vi "BRig_RT__Case_Exp__recordAnalogInput__PortC__netstream.vi"(0 "input_buffer_dataAnalog":u16[][](array[numeric]), 1 "input_index":i32, 2 "input_iOccurence":u16, 3 "resetOccurrence":bool, 4 "input_dataCurrent":u16[](array[numeric]), 5 "input_empytyArray":u16[](array[numeric]), 6 "input_iState_start":T1, 7 "input_fifo_hdl":refnum<k33>, 8 "input_iState_end":T1, 9 "input_fifo_error":errorcluster, 10 "input_AI1":i16, 12 "input_AI0":i16) -> (11 "output_fifo_hdl":refnum<k33>, 13 "error out":errorcluster, 14 "output_buffer_dataAnalog":u16[][](array[numeric]), 15 "output_index":i32, 16 "output_iOccurrence":u16)   [LabVIEW 2014]
uses:
  myRIO_BRig_RT__Case_Exp_stateList.ctl
panel:
  out "error out 2":errorcluster
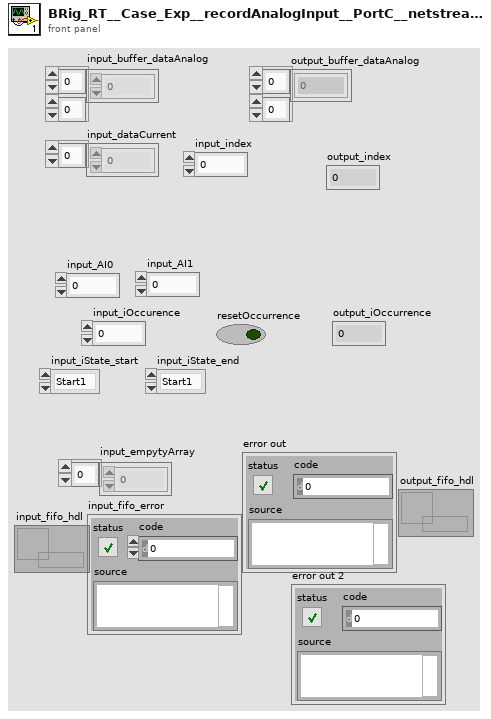
[diagram p1: front panel]
types:
  T1 = typedef "myRIO_BRig_RT__Case_Exp_stateList.ctl" = enum16{"Start1", "Start2", "Start3", "saveSettings1", "saveSettings2", "saveSettings3", "saveSettings4", "saveSettings_LC_ENL_l1", "saveSettings_LC_ENL_l2", "saveSettings_LC_Cue_l1", "saveSettings_LC_Cue_l2", "saveSettings6_LC_l1_Other", "SaveSettings6_LC_l2_Other", "setSettings_Audio", "setSettings_Laser", "initBlock_pre", "initBlock", "initBlock2", "initBlock_post", "initTrial_pre", "initTrial", "initTrial2", "initTrial3", "initTrial4", "initTrial_LC_ENL1", "initTrial_LC_Cue1", "initTrial_LC_Cue1_2", "initTrial_LC_Sel", "initTrial_post", "ENL1_pre", "ENL1", "ENL1_post", "ENL1Penalty_pre", "ENL1Penalty", "ENL2_pre", "ENL2", "ENL2Penalty_pre", "ENL2Penalty", "Cue1_pre", "Cue1", "Cue1_post", "Cue1Penalty_pre", "Cue1Penalty", "Cue2_pre", "Cue2", "Cue2Penalty_pre", "Cue2Penalty", "Selection_pre", "Selection", "Select_post", "SelectReward_pre", "SelectReward", "SelectRewardPost_pre", "SelectRewardPost", "SelectWrong_pre", "SelectWrong", "SelectWrong_post", "SelectTimeout_pre", "SelectTimeout", "SelectTimeout_post", "endTrial_pre", "endTrial1", "endTrial2", "endTrial3", "endTrial_post", "endBlock_pre", "endBlock", "endBlock_post", "endExp", "commConnect", "commUpload_pre", "commUpload_dataBlock", "commUpload_dataCurrent", "commUpload_dataExp", "commUpload_dataLC", "commUpload_dataTrial", "commUpload_post", "saveData_pre", "saveData_dataBlock", "saveData_dataCurrent", "saveData_dataExp", "saveData_dataLC", "saveData_dataTrial", "saveData_post", "empty_endBlock1", "empty_endBlock2", "empty_endTrial1", "empty_endTrial2", "empty_endTrial3", "empty_endTrial4", "empty_endTrial5", "dummyState", "dummyState_endBlock", "FreeReward_pre", "FreeReward", "FreeRewardPost_pre", "FreeRewardPost"}
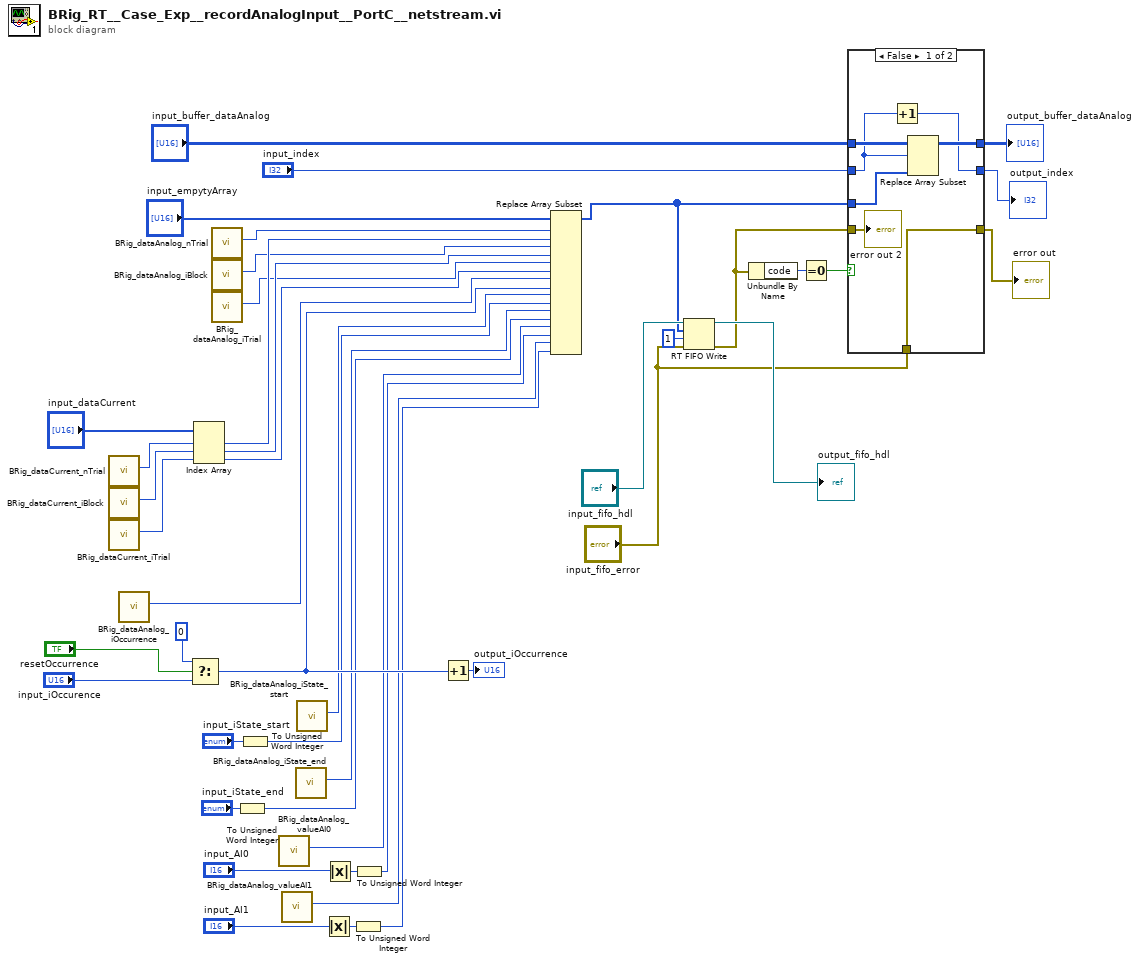
[diagram p0: block diagram]
diagram:
  n1 = call "BRig_dataCurrent_nTrial.vi"() -> ("output_nTrial"=w41:i32)  [unwired: 11 in]
  n2 = call "BRig_dataCurrent_iBlock.vi"() -> ("output_iBlock"=w40:i32)  [unwired: 11 in]
  n3 = call "BRig_dataCurrent_iTrial.vi"() -> ("output_iTrial"=w39:i32)  [unwired: 11 in]
  n4 = call "BRig_dataAnalog_iOccurrence.vi"() -> ("output_iOccurrence"=w22:i32)  [unwired: 11 in]
  n5 = Select(t=u16 0, s="resetOccurrence", f="input_iOccurence") -> (s? t:f=w21:u16)
  n6 = Index Array(array="input_dataCurrent", index #1=w41, index #2=w40, index #3=w39) -> (element #1=w27:u16, element #2=w25:u16, element #3=w23:u16)
  n7 = call "BRig_dataAnalog_nTrial.vi"() -> ("output_nTrial"=w28:i32)  [unwired: 11 in]
  n8 = call "BRig_dataAnalog_iBlock.vi"() -> ("output_iBlock"=w26:i32)  [unwired: 11 in]
  n9 = call "BRig_dataAnalog_iTrial.vi"() -> ("output_iTrial"=w24:i32)  [unwired: 11 in]
  n10 = To Unsigned Word Integer(number="input_iState_end") -> (unsigned 16bit integer=w17:u16)
  n11 = To Unsigned Word Integer(number="input_iState_start") -> (unsigned 16bit integer=w19:u16)
  n12 = call "BRig_dataAnalog_valueAI0.vi"() -> ("output_valueAI0"=w16:i32)  [unwired: 11 in]
  n13 = call "BRig_dataAnalog_valueAI1.vi"() -> ("output_valueAI1"=w14:i32)  [unwired: 11 in]
  n14 = call "BRig_dataAnalog_iState_end.vi"() -> ("output_iState_end"=w18:i32)  [unwired: 11 in]
  n15 = call "BRig_dataAnalog_iState_start.vi"() -> ("output_iState_start"=w20:i32)  [unwired: 11 in]
  n16 = Absolute Value(x="input_AI1") -> (abs(x)=w43:i16)
  n17 = Absolute Value(x="input_AI0") -> (abs(x)=w44:i16)
  n18 = To Unsigned Word Integer(number=w43) -> (unsigned 16bit integer=w13:u16)
  n19 = To Unsigned Word Integer(number=w44) -> (unsigned 16bit integer=w15:u16)
  n20 = Increment(x=w21) -> (x+1=→"output_iOccurrence":u16)
  n21 = Replace Array Subset(array="input_empytyArray", new element #1=w27, index #1=w28, new element #2=w25, index #2=w26, new element #3=w23, index #3=w24, new element #4=w21, index #4=w22, new element #5=w19, index #5=w20, new element #6=w17, index #6=w18, new element #7=w15, index #7=w16, new element #8=w13, index #8=w14) -> (w5:u16[])
  n22 = RT FIFO Write(0:"input_fifo_hdl", 1:w5, 2:1 ("timeout in ms (0)"), 3:"input_fifo_error") -> (8:→"output_fifo_hdl":refnum<k33>, 11:w3:errorcluster)  [unwired: 1 in, 2 out]
  n23 = Unbundle By Name(w3) -> ("code"=w30:i32)
  n24 = Equal To 0?(x=w30) -> (x = 0?=w12:bool)
  n25 = case shown="False" w12 {
    tunnel: "input_buffer_dataAnalog" -> [w51 w54]
    tunnel: "input_index" -> [w48 w53]
    tunnel: [w50 w54] -> w10
    tunnel: [w47 w53] -> w9
    tunnel: w5 -> [w49 _]
    tunnel: w3 -> [w45 w52]
    tunnel: [w46 w52] -> w8
    tunnel: "input_fifo_error" -> [w46 _]
    frame False {
      n26 = Increment(x=w48) -> (x+1=w47:i32)
      n27 = Replace Array Subset(array=w51, new element=w49, index (row)=w48) -> (w50:u16[][])  [unwired: 1 in]
      "error out 2" <- w45
    }
    frame True {
    }
  }
  "output_buffer_dataAnalog" <- w10
  "output_index" <- w9
  "error out" <- w8
